vi "Actor Core.vi"(8 "error in":errorcluster, 11 "WS Test Server in":refnum<class "WS Server Subscriber.lvclass">) -> (0 "error out":errorcluster, 3 "Actor out":refnum<class "Actor.lvclass">)   [LabVIEW 2021, in "Secure Echo Broadcast With Server Manager.lvlib" / "WS Server Subscriber.lvclass"]
doc: "(<B>Filename</B>: Actor Framework.lvlib:Actor.lvclass:Actor Core.vi)\n\nReceives messages to the actor, reacts to them, and initiates any error handling that may shut the actor down.\n\nDescendant classes may override this VI to append parallel tasks for the actor to complete while it handles messages. Overrides use the Call Parent Method node."
uses:
  WS Server Subscriber.lvclass
  C:/Program Files/National Instruments/LabVIEW 2021/vi.lib/ActorFramework/Actor/Actor.lvclass
  <vilib>/ActorFramework/Actor/Actor.lvclass
  WebSocket Actor/WebSocket Server/typedefs/Listener Settings.ctl
  WS Server Subscriber Messages/WebSocket Server Enqueuer Msg/WebSocket Server Enqueuer Msg.lvclass
  C:/Projects/WebSocket-Actor/WebSocket Actor/Abstract Messages/WebSocket Server-Service Enqueuer Msg/WebSocket Server-Service Enqueuer Msg.lvclass
  <vilib>/ActorFramework/Message Enqueuer/Message Enqueuer.lvclass
  <vilib>/ActorFramework/Actor/Actor.lvclass/Actor.ctl
  <vilib>/ActorFramework/Message Enqueuer/Message Enqueuer.lvclass/Message Enqueuer.ctl
  WS Server Subscriber.lvclass/WS Server Subscriber.ctl
  25efce69-9ab1-4e82-b2fb-50220ea39495.vi
  <vilib>/ActorFramework/Message Enqueuer/Init from Existing Queue.vi
  WebSocket Actor/WebSocket Server Manager Messages/Launch Server Msg/Launch Server Msg.lvclass
  WebSocket Actor/WebSocket Server/WebSocket Server.lvclass
  <userlib>/_OpenG.lib/error/error.llb/openg_error.lvlib
  WS Server Subscriber Messages/Send Packets Msg/Send Packets Msg.lvclass
  C:/Projects/WebSocket-Actor/Examples/Secure Echo Broadcast With Server Manager/WS Server Subscriber/WS Server Subscriber.lvclass
  C:/Program Files/National Instruments/LabVIEW 2021/vi.lib/ActorFramework/Message/Message.lvclass
  C:/Projects/WebSocket-Actor/Examples/Secure Echo Broadcast With Server Manager/WS Server Subscriber Messages/WebSocket Server Enqueuer Msg/WebSocket Server Enqueuer Msg.lvclass
panel:
  in  "Send Period (ms)":i32=1000
  in  "Number of Packets":i32=1
  in  "Send":bool
  in  "Data To Send":string
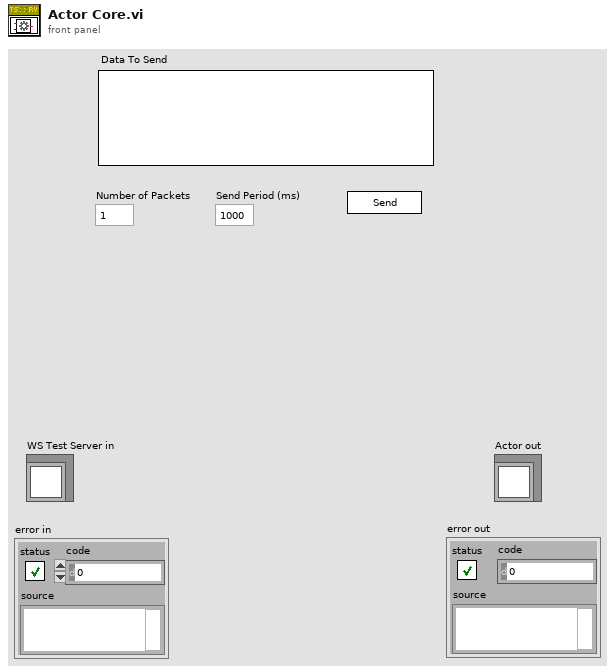
[diagram p1: front panel]
types:
  T1 = enum8{"Enabled", "Disabled", "Disabled and Grayed Out"}
  T2 = typedef "WebSocket Actors.lvlib/WebSocket Server.lvclass/Listener Settings.ctl" = cluster{"resolve remote address (T)":bool, "timeout ms (-1)":i32, "net address":u32, "port":u16}
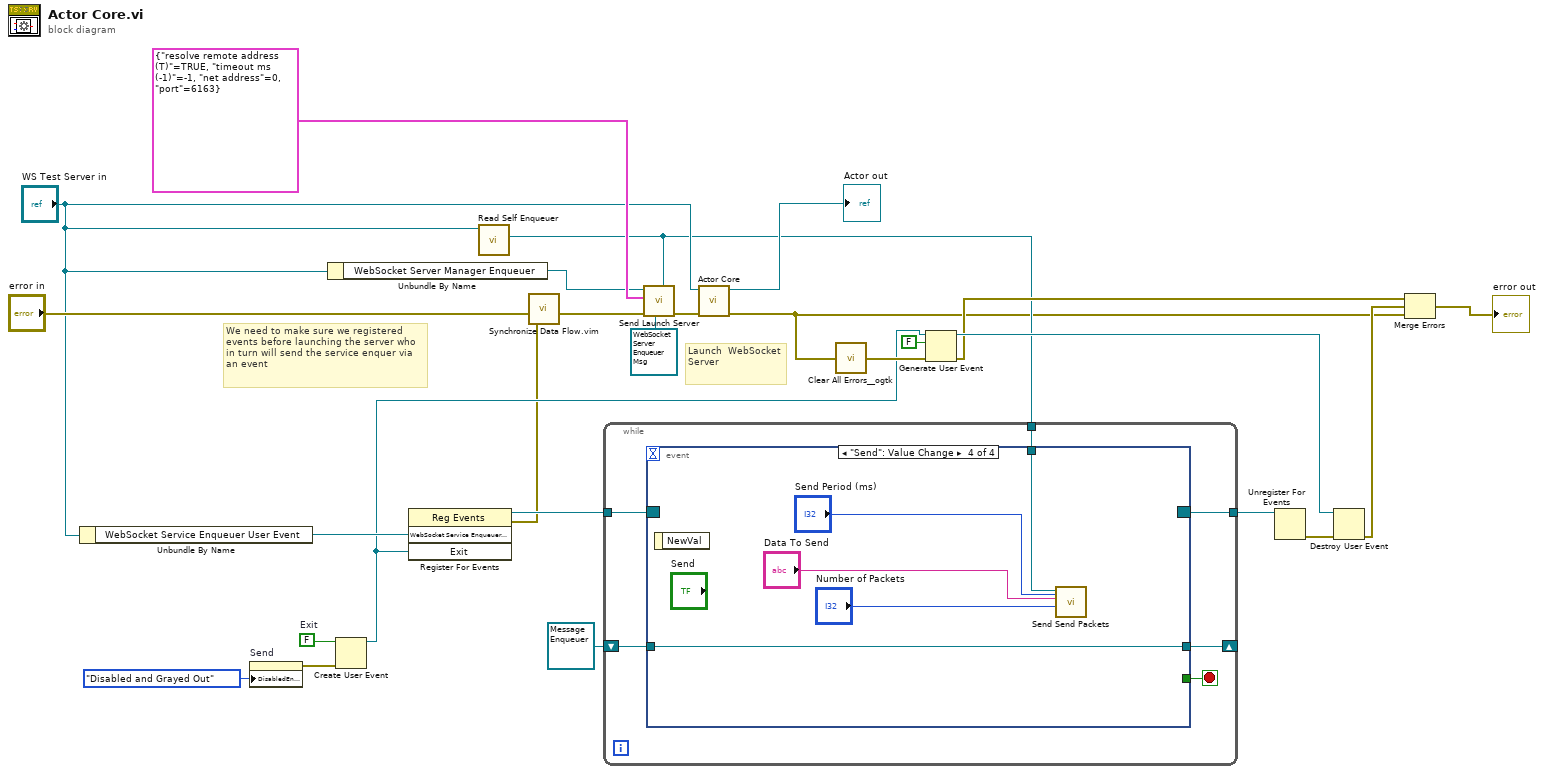
[diagram p0: block diagram]
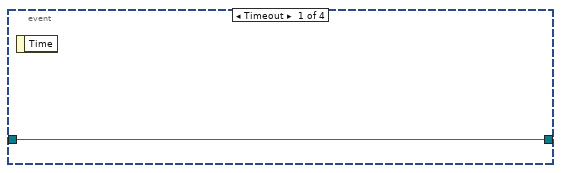
[diagram p2: hidden frame]
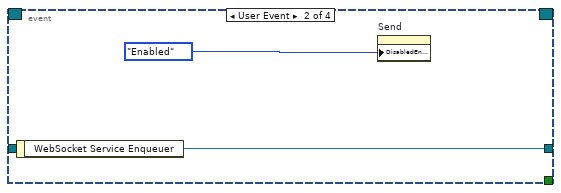
[diagram p3: hidden frame]
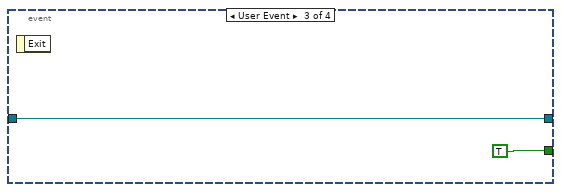
[diagram p4: hidden frame]
diagram:
  w17 = FALSE  # Exit
  # "We need to make sure we registered events before launching the server who in turn will send the service enquer via an event"
  # "Launch  WebSocket Server"
  n1 = Unbundle By Name("WS Test Server in") -> ("WebSocket Service Enqueuer User Event"=w19:refnum<user-event>)
  n2 = property on="Send" class="Bool"("DisabledEnum"=T1."Disabled and Grayed Out" ("Disabled")) -> (error out=w6:errorcluster)  [unwired: 2 in, 1 out]
  n3 = Unbundle By Name("WS Test Server in") -> ("WebSocket Server Manager Enqueuer"=w22:refnum<class "Message Enqueuer.lvclass">)
  n4 = Create User Event(user event datatype=w17, error in=w6) -> (user event=w14:refnum<user-event>)  [unwired: 1 out]
  n5 = register-events(w19, w14) -> (reference out=w18:refnum<event-registration>, error out=w1:errorcluster)  [unwired: 2 in]
  n6 = call <vilib>:"Read Self Enqueuer.vi"("Actor"="WS Test Server in") -> ("Self Enqueuer"=w4:refnum<class "Message Enqueuer.lvclass">)  [unwired: 10 in]
  n7 = call "Synchronize Data Flow.vim"("input 4"=w1, "input 3"="error in") -> ("output 3"=w2:errorcluster)  [unwired: 2 in, 3 out]
  n8 = while {
    tunnel: w18 -> [w32]
    shift-right: [w30] -> _
    shift-left: refnum<class "Message Enqueuer.lvclass"> refnum ("WebSocket Service Enqueuer") -> [w29]
    tunnel: [w28] -> w13
    tunnel: w4 -> [w27]
    stop <- w31 stop-if-true
    n9 = event shown="[3] \"Send\": Value Change" {
      selector: w32 -> [_ _ _ _]
      dyn-events: [_ _ _ _] -> w28
      timeout: _ -> [_ _ _ _]
      tunnel: [_ _ TRUE _] -> w31
      tunnel: [w33 w35 w36 w42] -> w30
      tunnel: w29 -> [w33 _ w36 w42]
      tunnel: w27 -> [_ _ _ w41]
      event Timeout {
        n10 = event-data() -> ()  [unwired: 1 in, 1 out]
      }
      event User Event {
        n11 = event-data() -> ("WebSocket Service Enqueuer"=w35:refnum<class "Message Enqueuer.lvclass">)  [unwired: 1 in]
        n12 = property on="Send" class="Bool"("DisabledEnum"=T1."Enabled" ("Disabled")) -> ()  [unwired: 2 in, 2 out]
      }
      event User Event {
        n13 = event-data() -> ()  [unwired: 1 in, 1 out]
      }
      event "Send": Value Change {
        n14 = event-data() -> ()  [unwired: 1 in, 1 out]
        n15 = call "Send Send Packets.vi"("Send Period (ms)"="Send Period (ms)", "Number of Packets"="Number of Packets", "Data To Send"="Data To Send", "Message Enqueuer in"=w41) -> ()  [unwired: 6 in, 2 out]
      }
    }
  }
  n16 = call "Send Launch Server.vi"("Subscriber Enqueuer"=w4, "Receive Server Enqueuer Handler"=refnum<class "WebSocket Server Enqueuer Msg.lvclass"> refnum ("Echo Broadcast Test With Server Manager.lvlib:WebSocket Server Enqueuer Msg.lvclass"), "error in (no error)"=w2, "Listener Settings"=T2 {"resolve remote address (T)"=TRUE, "timeout ms (-1)"=-1, "net address"=0, "port"=6163}, "Message Enqueuer in"=w22) -> ("error out"=w23:errorcluster)  [unwired: 5 in, 1 out]
  n17 = call-parent "Actor Core.vi"("error in"=w23, "Actor in"="WS Test Server in") -> ("error out"=w3:errorcluster, "Actor out"=→"Actor out":refnum<class "Actor.lvclass">)  [unwired: 8 in]
  n18 = call <userlib>:"Clear All Errors__ogtk.vi"("Error In"=w3) -> ("Error Out"=w15:errorcluster)  [unwired: 3 in]
  n19 = Generate User Event(user event=w14, event data cluster=FALSE ("event data"), error in=w15) -> (user event out=w11:refnum<user-event>, error out=w8:errorcluster)  [unwired: 1 in]
  n20 = Unregister For Events(event registration refnum=w13) -> (error out=w12:errorcluster)  [unwired: 1 in]
  n21 = Destroy User Event(user event=w11, error in=w12) -> (error out=w9:errorcluster)
  n22 = Merge Errors(w8, w9, w3) -> (→"error out":errorcluster)
